vi "QX_guanli.vi"(4 "key":string, 6 "quanx":string, 7 "LabVIEW Web Service Request":refnum<class "Web Request.lvclass"> caption="LabVIEW Web服务请求", 8 "id":string, 9 "action":string, 10 "values":string, 11 "juese":string) -> (0 "error":errorcluster)   [LabVIEW 2017]
uses:
  <vilib>/wsapi/Web Request.lvclass
panel:
  out "postdata":string caption="post数据"
  out "error out":errorcluster caption="错误输出"
  # "Web服务请求输入接线端用于调用“Web服务”选板的VI。除非不需要访问该选板，否则不要在连线板上删除这个输入接线端。"
  # "添加至连线板的每一个其他输入控件，在URL中对应于一个输入。如需在接线端模式输出（默认设置）下包含显示控件，则该显示控件必须与连线板相连。"
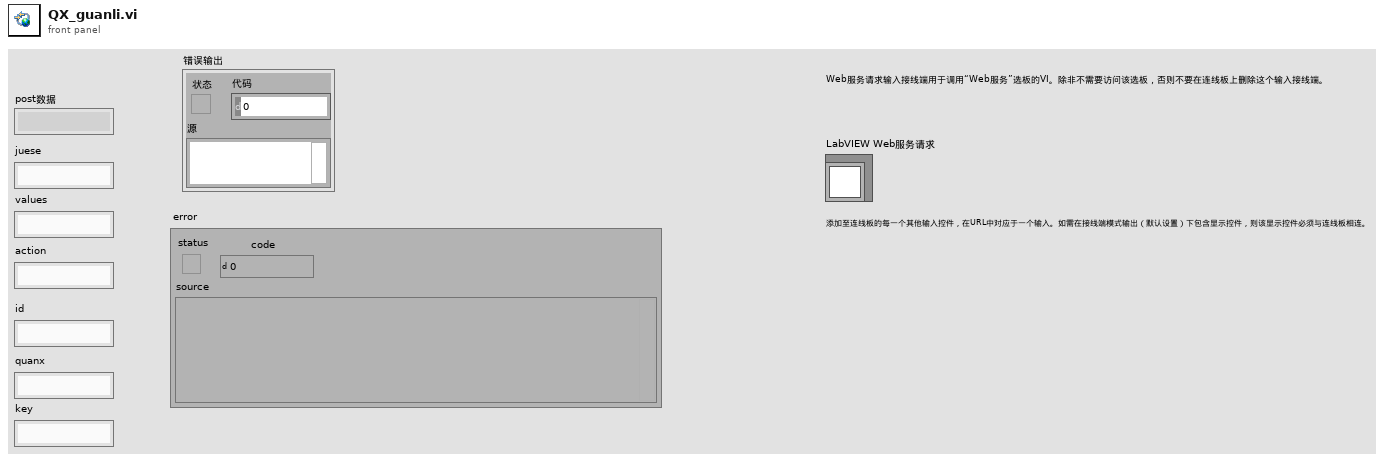
[diagram p1: front panel]
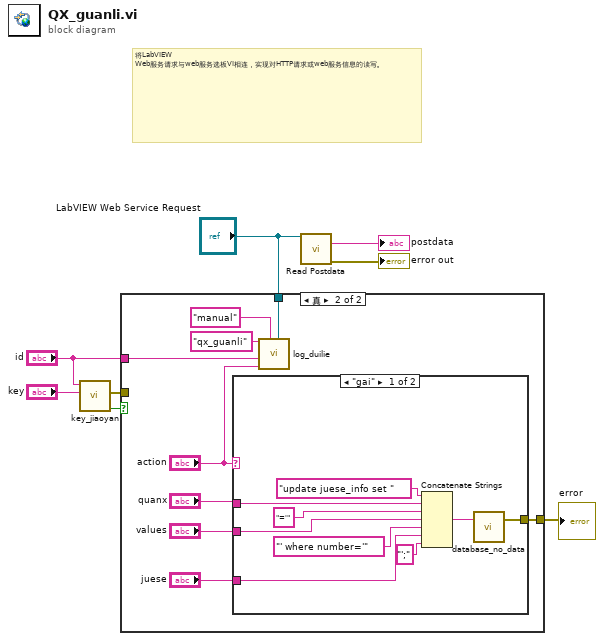
[diagram p0: block diagram]
diagram:
  # "将LabVIEW Web服务请求与web服务选板VI相连，实现对HTTP请求或web服务信息的读写。"
  n1 = call "key_jiaoyan.vi"("key_client"="key", "gonghao"="id") -> ("jy"=w3:bool, "error"=w2:errorcluster)  [unwired: 8 in]
  n2 = case shown="真" w3 {
    tunnel: [w9 w18] -> w7
    tunnel: "LabVIEW Web Service Request" -> [_ w14]
    tunnel: "id" -> [_ w10]
    tunnel: w2 -> [w9 _]
    frame False {
    }
    frame True {
      n3 = case shown="\"gai\"" "action" {
        tunnel: [w26 _] -> w18
        tunnel: "quanx" -> [w22 _]
        tunnel: "values" -> [w20 _]
        tunnel: "juese" -> [w25 _]
        frame "gai" {
          n4 = Concatenate Strings("update juese_info set " ("格式字符串"), w22, "='" ("格式字符串"), w20, "' where number='" ("字符串"), w25, "';" ("字符串")) -> (w27:string)
          n5 = call "database_no_data.vi"("input"=w27) -> ("error"=w26:errorcluster)  [unwired: 2 in]
        }
        frame Default {
        }
      }
      n6 = call "log_duilie.vi"("LabVIEW Web Service Request"=w14, "type"="manual", "action"="action", "user"=w10, "yw"="qx_guanli") -> ()  [unwired: 7 in]
    }
  }
  "error" <- w7
  n7 = call <vilib>:"Read Postdata.vi"("LabVIEW Web Service Request"="LabVIEW Web Service Request") -> ("postdata"=→"postdata":string, "error out"=→"error out":errorcluster)  [unwired: 12 in, 1 out]
